vi "write counter.vi"() -> (2 "Counter 2":u16=1, 3 "State Machine out":refnum<class "CCS_State Machine.lvclass">)   [LabVIEW 2018]
uses:
  State Machine/CCS_State Machine.lvclass
  State Machine/CCS_State Machine.lvclass/CCS_State Machine.ctl
panel:
  in  "State Machine.lvclass":refnum<class "CCS_State Machine.lvclass">
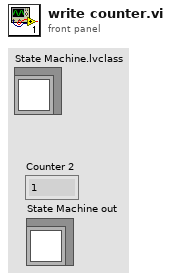
[diagram p1: front panel]
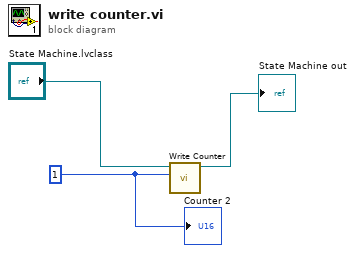
[diagram p0: block diagram]
diagram:
  w1 = u16 1 ("Counter")
  n1 = call "Write Counter.vi"("Counter"=w1, "State Machine in"="State Machine.lvclass") -> ("State Machine out"=→"State Machine out":refnum<class "CCS_State Machine.lvclass">)  [unwired: 8 in, 1 out]
  "Counter 2" <- w1
